vi "Send Update Preview Image.vi"(8 "error in (no error)":errorcluster, 9 "Image":refnum<data-value>, 10 "Draw Offset":T1, 11 "UI in":refnum<class "UI.lvclass">) -> (0 "error out":errorcluster)   [LabVIEW 2020, in "AR Example.lvlib" / "UI.lvclass"]
uses:
  UI.lvclass
  g_ar_toolkit.image/Image Draw Offset.ctl
  Update Preview Event.ctl
  UI.lvclass/UI.ctl
  g_ar_toolkit.image/g_ar_toolkit.image.lvlib
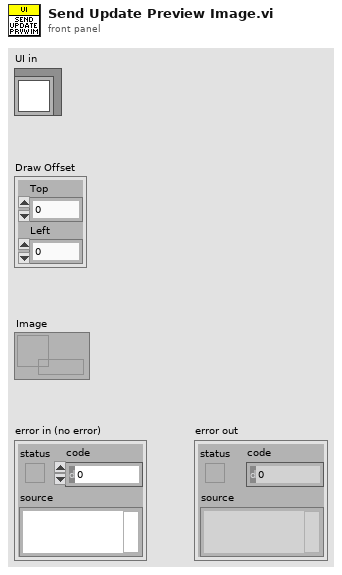
[diagram p1: front panel]
types:
  T1 = typedef "g_ar_toolkit.image.lvlib/Image Draw Offset.ctl" = cluster{"Top":i16, "Left":i16}
  T2 = typedef "AR Example.lvlib/UI.lvclass/Update Preview Event.ctl" = cluster{"Image":refnum<data-value>, "Draw Offset":T1}
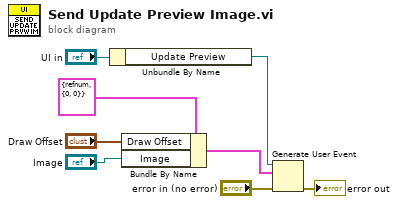
[diagram p0: block diagram]
diagram:
  n1 = Unbundle By Name("UI in") -> ("Update Preview"=w7:refnum<user-event>)
  n2 = Bundle By Name(cluster=T2 {"Image"=refnum, "Draw Offset"={"Top"=0, "Left"=0}} ("event data"), "Draw Offset"="Draw Offset", "Image"="Image") -> (w3:T2)
  n3 = Generate User Event(user event=w7, event data cluster=w3, error in="error in (no error)") -> (error out=→"error out":errorcluster)  [unwired: 1 in, 1 out]
